vi "BCU诊断标定.vi"(8 "CAN端口":u16(ring), 9 "设备索引号":u16(ring), 10 "CAN卡类型":u32(ring)=21, 11 "Myindex":dbl=1.0) -> (3 "成功":bool)   [LabVIEW 2013] (continued)
                n960 = property on="从板个数" class="DigNum (严格)"("NumText.BGColor"=u32 13816530) -> ()  [unwired: 2 in, 2 out]
                n961 = Select(t=0, s=w1284, f=1) -> (s? t:f=w1283:i32)
                n962 = property on="项目信息" class="Tbl (严格)"("Disabled"=w1283) -> ()  [unwired: 2 in, 2 out]
                n963 = global read "功能码全局.vi" "主板项目信息5"() -> (w1291:bool[])
                n964 = global read "功能码全局.vi" "主板项目信息6"() -> (w1289:bool[])
                n965 = Index Array(array=w1291, index=4 ("索引")) -> (element=w1287:bool)
                n966 = Index Array(array=w1289, index=5 ("索引")) -> (element=w1288:bool)
                n967 = Not(x=w1297) -> (.not. x?=w1296:bool)
              }
              frame "温度起始值" {
                w1333 = 2
                w1335 = FALSE
                n968 = property on="电池实际容量(A)" class="DigNum (严格)"("Disabled"=w1333) -> ()  [unwired: 2 in, 2 out]
                n969 = property on="使用者" class="DigNum (严格)"("Disabled"=w1333) -> ()  [unwired: 2 in, 2 out]
                n970 = property on="SOH(%)" class="DigNum (严格)"("Disabled"=w1333) -> ()  [unwired: 2 in, 2 out]
                n971 = property on="电池额定容量(A)" class="DigNum (严格)"("Disabled"=w1333) -> ()  [unwired: 2 in, 2 out]
                n972 = property on="SOC(%)" class="DigNum (严格)"("Disabled"=w1333) -> ()  [unwired: 2 in, 2 out]
                n973 = local read "从板个数"() -> (w1331:dbl)
                n974 = property on="系统时钟" class="Str"("Disabled"=w1333) -> ()  [unwired: 2 in, 2 out]
                n975 = property on="配置文件版本" class="Str"("Disabled"=w1333) -> ()  [unwired: 2 in, 2 out]
                n976 = property on="车架(牌)号" class="Str"("Disabled"=w1333) -> ()  [unwired: 2 in, 2 out]
                n977 = property on="产品编号" class="Str"("Disabled"=w1333) -> ()  [unwired: 2 in, 2 out]
                n978 = control-ref of="项目信息"() -> (w1332:refnum<vi>)
                n979 = stacked-sequence {
                  tunnel: w1332 -> [w1344 w1347 w1360]
                  tunnel: w1331 -> [w1337 w1346 w1359]
                  frame #0 {
                    n980 = Multiply(x=w1337, y=3.0) -> (x*y=w1339:dbl)
                    n981 = Compound Arithmetic op=ADD(23.0 ("值"), w1339) -> (w1341:dbl)
                    n982 = Bundle(w1341, 0) -> (w1343:cluster{dbl, i32})  [unwired: 1 out]
                    n983 = property class="Tbl (严格)"(reference=w1344, "Index Values"=w1343) -> ()  [unwired: 1 in, 2 out]
                  }
                  frame #1 {
                    n984 = for {
                      N: 10 -> [_]
                      tunnel: w1347 -> [w1357]
                      tunnel: w1346 -> [w1352]
                      i -> [w1351]
                      n985 = Multiply(x=4.0, y=w1352) -> (x*y=w1349:dbl)
                      n986 = Compound Arithmetic op=ADD(24.0 ("值"), w1349, w1351) -> (w1354:dbl)
                      n987 = Bundle(w1354, 0) -> (w1356:cluster{dbl, i32})  [unwired: 1 out]
                      n988 = property class="Tbl (严格)"(reference=w1357, "Active Cell"=w1356, "Cell BG Color"=u32 16448250) -> ()  [unwired: 1 in, 2 out]
                    }
                  }
                  frame #2 {
                    n989 = Increment(x=w1359) -> (x+1=w1358:dbl)
                    n990 = for {
                      N: w1358 -> [_]
                      tunnel: w1360 -> [w1370]
                      tunnel: w1359 -> [w1365]
                      i -> [w1364]
                      n991 = Multiply(x=3.0, y=w1365) -> (x*y=w1362:dbl)
                      n992 = Compound Arithmetic op=ADD(23.0 ("值"), w1362, w1364) -> (w1367:dbl)
                      n993 = Bundle(w1367, 0) -> (w1369:cluster{dbl, i32})  [unwired: 1 out]
                      n994 = property class="Tbl (严格)"(reference=w1370, "Active Cell"=w1369, "Cell BG Color"=u32 6618880) -> ()  [unwired: 1 in, 2 out]
                    }
                  }
                }
                n995 = Select(t=0, s=w1322, f=1) -> (s? t:f=w1321:i32)
                n996 = property on="从板个数" class="DigNum (严格)"("NumText.BGColor"=u32 13816530) -> ()  [unwired: 2 in, 2 out]
                n997 = property on="项目信息" class="Tbl (严格)"("Disabled"=w1321) -> ()  [unwired: 2 in, 2 out]
                n998 = global read "功能码全局.vi" "主板项目信息5"() -> (w1329:bool[])
                n999 = global read "功能码全局.vi" "主板项目信息6"() -> (w1327:bool[])
                n1000 = Index Array(array=w1329, index=5 ("索引")) -> (element=w1326:bool)
                n1001 = Index Array(array=w1327, index=6 ("索引")) -> (element=w1325:bool)
                n1002 = Not(x=w1335) -> (.not. x?=w1334:bool)
              }
              frame "保险位置" {
                w1383 = 2
                w1385 = FALSE
                n1003 = property on="电池实际容量(A)" class="DigNum (严格)"("Disabled"=w1383) -> ()  [unwired: 2 in, 2 out]
                n1004 = property on="使用者" class="DigNum (严格)"("Disabled"=w1383) -> ()  [unwired: 2 in, 2 out]
                n1005 = property on="SOH(%)" class="DigNum (严格)"("Disabled"=w1383) -> ()  [unwired: 2 in, 2 out]
                n1006 = property on="电池额定容量(A)" class="DigNum (严格)"("Disabled"=w1383) -> ()  [unwired: 2 in, 2 out]
                n1007 = property on="SOC(%)" class="DigNum (严格)"("Disabled"=w1383) -> ()  [unwired: 2 in, 2 out]
                n1008 = local read "从板个数"() -> (w1381:dbl)
                n1009 = property on="系统时钟" class="Str"("Disabled"=w1383) -> ()  [unwired: 2 in, 2 out]
                n1010 = property on="配置文件版本" class="Str"("Disabled"=w1383) -> ()  [unwired: 2 in, 2 out]
                n1011 = property on="车架(牌)号" class="Str"("Disabled"=w1383) -> ()  [unwired: 2 in, 2 out]
                n1012 = property on="产品编号" class="Str"("Disabled"=w1383) -> ()  [unwired: 2 in, 2 out]
                n1013 = control-ref of="项目信息"() -> (w1382:refnum<vi>)
                n1014 = stacked-sequence {
                  tunnel: w1382 -> [w1394 w1397]
                  tunnel: w1381 -> [w1387 w1396]
                  frame #0 {
                    n1015 = Multiply(x=w1387, y=4.0) -> (x*y=w1389:dbl)
                    n1016 = Compound Arithmetic op=ADD(24.0 ("值"), w1389) -> (w1391:dbl)
                    n1017 = Bundle(w1391, 0) -> (w1393:cluster{dbl, i32})  [unwired: 1 out]
                    n1018 = property class="Tbl (严格)"(reference=w1394, "Index Values"=w1393) -> ()  [unwired: 1 in, 2 out]
                  }
                  frame #1 {
                    n1019 = for {
                      N: 20 -> [_]
                      tunnel: w1397 -> [w1407]
                      tunnel: w1396 -> [w1402]
                      i -> [w1401]
                      n1020 = Multiply(x=4.0, y=w1402) -> (x*y=w1399:dbl)
                      n1021 = Compound Arithmetic op=ADD(24.0 ("值"), w1399, w1401) -> (w1404:dbl)
                      n1022 = Bundle(w1404, 0) -> (w1406:cluster{dbl, i32})  [unwired: 1 out]
                      n1023 = property class="Tbl (严格)"(reference=w1407, "Active Cell"=w1406, "Cell BG Color"=u32 6618880) -> ()  [unwired: 1 in, 2 out]
                    }
                  }
                }
                n1024 = property on="从板个数" class="DigNum (严格)"("NumText.BGColor"=u32 13816530) -> ()  [unwired: 2 in, 2 out]
                n1025 = Select(t=0, s=w1374, f=1) -> (s? t:f=w1372:i32)
                n1026 = global read "功能码全局.vi" "主板项目信息4"() -> (w1379:bool[])
                n1027 = property on="项目信息" class="Tbl (严格)"("Disabled"=w1372) -> ()  [unwired: 2 in, 2 out]
                n1028 = Index Array(array=w1379, index #1=5 ("索引"), index #2=6 ("索引")) -> (element #1=w1377:bool, element #2=w1376:bool)
                n1029 = Not(x=w1385) -> (.not. x?=w1384:bool)
              }
              frame "SOC" {
                w1418 = 2
                w1420 = FALSE
                n1030 = property on="电池实际容量(A)" class="DigNum (严格)"("Disabled"=w1418) -> ()  [unwired: 2 in, 2 out]
                n1031 = property on="使用者" class="DigNum (严格)"("Disabled"=w1418) -> ()  [unwired: 2 in, 2 out]
                n1032 = property on="SOH(%)" class="DigNum (严格)"("Disabled"=w1418) -> ()  [unwired: 2 in, 2 out]
                n1033 = property on="电池额定容量(A)" class="DigNum (严格)"("Disabled"=w1418) -> ()  [unwired: 2 in, 2 out]
                n1034 = property on="从板个数" class="DigNum (严格)"("NumText.BGColor"=u32 13816530) -> ()  [unwired: 2 in, 2 out]
                n1035 = property on="系统时钟" class="Str"("Disabled"=w1418) -> ()  [unwired: 2 in, 2 out]
                n1036 = property on="配置文件版本" class="Str"("Disabled"=w1418) -> ()  [unwired: 2 in, 2 out]
                n1037 = property on="车架(牌)号" class="Str"("Disabled"=w1418) -> ()  [unwired: 2 in, 2 out]
                n1038 = property on="项目信息" class="Tbl (严格)"("Disabled"=w1418) -> ()  [unwired: 2 in, 2 out]
                n1039 = property on="产品编号" class="Str"("Disabled"=w1418) -> ()  [unwired: 2 in, 2 out]
                n1040 = Select(t=0, s=w1410, f=0) -> (s? t:f=w1409:i32)
                n1041 = property on="SOC(%)" class="DigNum (严格)"("Disabled"=w1409) -> ()  [unwired: 2 in, 2 out]
                n1042 = property on="项目信息2" class="Clust (严格)"("DisabledEnum"=w1409) -> ()  [unwired: 2 in, 2 out]
                n1043 = global read "功能码全局.vi" "主板项目信息7"() -> (w1416:bool[])
                n1044 = Index Array(array=w1416, index #1=2 ("索引"), index #2=5 ("索引")) -> (element #1=w1414:bool, element #2=w1413:bool)
                n1045 = Not(x=w1420) -> (.not. x?=w1419:bool)
              }
              frame "电池额定实际容量" {
                w1432 = 2
                w1434 = FALSE
                n1046 = property on="使用者" class="DigNum (严格)"("Disabled"=w1432) -> ()  [unwired: 2 in, 2 out]
                n1047 = property on="SOH(%)" class="DigNum (严格)"("Disabled"=w1432) -> ()  [unwired: 2 in, 2 out]
                n1048 = property on="SOC(%)" class="DigNum (严格)"("Disabled"=w1432) -> ()  [unwired: 2 in, 2 out]
                n1049 = property on="从板个数" class="DigNum (严格)"("NumText.BGColor"=u32 13816530) -> ()  [unwired: 2 in, 2 out]
                n1050 = property on="系统时钟" class="Str"("Disabled"=w1432) -> ()  [unwired: 2 in, 2 out]
                n1051 = property on="配置文件版本" class="Str"("Disabled"=w1432) -> ()  [unwired: 2 in, 2 out]
                n1052 = property on="车架(牌)号" class="Str"("Disabled"=w1432) -> ()  [unwired: 2 in, 2 out]
                n1053 = property on="项目信息" class="Tbl (严格)"("Disabled"=w1432) -> ()  [unwired: 2 in, 2 out]
                n1054 = property on="产品编号" class="Str"("Disabled"=w1432) -> ()  [unwired: 2 in, 2 out]
                n1055 = Select(t=0, s=w1424, f=1) -> (s? t:f=w1423:i32)
                n1056 = property on="电池实际容量(A)" class="DigNum (严格)"("Disabled"=w1423) -> ()  [unwired: 2 in, 2 out]
                n1057 = property on="电池额定容量(A)" class="DigNum (严格)"("Disabled"=w1423) -> ()  [unwired: 2 in, 2 out]
                n1058 = property on="项目信息2" class="Clust (严格)"("DisabledEnum"=w1423) -> ()  [unwired: 2 in, 2 out]
                n1059 = global read "功能码全局.vi" "主板项目信息7"() -> (w1430:bool[])
                n1060 = Index Array(array=w1430, index #1=3 ("索引"), index #2=6 ("索引")) -> (element #1=w1428:bool, element #2=w1427:bool)
                n1061 = Not(x=w1434) -> (.not. x?=w1433:bool)
              }
              frame "配置文件版本" {
                w1447 = 2
                w1449 = FALSE
                n1062 = property on="使用者" class="DigNum (严格)"("Disabled"=w1447) -> ()  [unwired: 2 in, 2 out]
                n1063 = property on="SOH(%)" class="DigNum (严格)"("Disabled"=w1447) -> ()  [unwired: 2 in, 2 out]
                n1064 = property on="SOC(%)" class="DigNum (严格)"("Disabled"=w1447) -> ()  [unwired: 2 in, 2 out]
                n1065 = property on="电池实际容量(A)" class="DigNum (严格)"("Disabled"=w1447) -> ()  [unwired: 2 in, 2 out]
                n1066 = property on="从板个数" class="DigNum (严格)"("NumText.BGColor"=u32 13816530) -> ()  [unwired: 2 in, 2 out]
                n1067 = property on="电池额定容量(A)" class="DigNum (严格)"("Disabled"=w1447) -> ()  [unwired: 2 in, 2 out]
                n1068 = property on="系统时钟" class="Str"("Disabled"=w1447) -> ()  [unwired: 2 in, 2 out]
                n1069 = property on="车架(牌)号" class="Str"("Disabled"=w1447) -> ()  [unwired: 2 in, 2 out]
                n1070 = property on="项目信息" class="Tbl (严格)"("Disabled"=w1447) -> ()  [unwired: 2 in, 2 out]
                n1071 = property on="产品编号" class="Str"("Disabled"=w1447) -> ()  [unwired: 2 in, 2 out]
                n1072 = Select(t=0, s=w1438, f=1) -> (s? t:f=w1437:i32)
                n1073 = property on="项目信息2" class="Clust (严格)"("DisabledEnum"=w1437) -> ()  [unwired: 2 in, 2 out]
                n1074 = property on="配置文件版本" class="Str"("Disabled"=w1437) -> ()  [unwired: 2 in, 2 out]
                n1075 = global read "功能码全局.vi" "主板项目信息5"() -> (w1445:bool[])
                n1076 = global read "功能码全局.vi" "主板项目信息6"() -> (w1444:bool[])
                n1077 = Index Array(array=w1445, index=6 ("索引")) -> (element=w1442:bool)
                n1078 = Index Array(array=w1444, index=7 ("索引")) -> (element=w1441:bool)
                n1079 = Not(x=w1449) -> (.not. x?=w1448:bool)
              }
              frame "参数修改记录" {
                w1462 = 2
                w1464 = FALSE
                n1080 = property on="SOH(%)" class="DigNum (严格)"("Disabled"=w1462) -> ()  [unwired: 2 in, 2 out]
                n1081 = property on="SOC(%)" class="DigNum (严格)"("Disabled"=w1462) -> ()  [unwired: 2 in, 2 out]
                n1082 = property on="电池实际容量(A)" class="DigNum (严格)"("Disabled"=w1462) -> ()  [unwired: 2 in, 2 out]
                n1083 = property on="电池额定容量(A)" class="DigNum (严格)"("Disabled"=w1462) -> ()  [unwired: 2 in, 2 out]
                n1084 = property on="从板个数" class="DigNum (严格)"("NumText.BGColor"=u32 13816530) -> ()  [unwired: 2 in, 2 out]
                n1085 = property on="系统时钟" class="Str"("Disabled"=w1462) -> ()  [unwired: 2 in, 2 out]
                n1086 = property on="车架(牌)号" class="Str"("Disabled"=w1462) -> ()  [unwired: 2 in, 2 out]
                n1087 = property on="配置文件版本" class="Str"("Disabled"=w1462) -> ()  [unwired: 2 in, 2 out]
                n1088 = property on="项目信息" class="Tbl (严格)"("Disabled"=w1462) -> ()  [unwired: 2 in, 2 out]
                n1089 = property on="产品编号" class="Str"("Disabled"=w1462) -> ()  [unwired: 2 in, 2 out]
                n1090 = Select(t=0, s=w1453, f=1) -> (s? t:f=w1452:i32)
                n1091 = property on="使用者" class="DigNum (严格)"("Disabled"=w1452) -> ()  [unwired: 2 in, 2 out]
                n1092 = property on="项目信息2" class="Clust (严格)"("DisabledEnum"=w1452) -> ()  [unwired: 2 in, 2 out]
                n1093 = global read "功能码全局.vi" "主板项目信息7"() -> (w1459:bool[])
                n1094 = global read "功能码全局.vi" "主板项目信息5"() -> (w1460:bool[])
                n1095 = Index Array(array=w1459, index=0 ("索引")) -> (element=w1457:bool)
                n1096 = Index Array(array=w1460, index=7 ("索引")) -> (element=w1456:bool)
                n1097 = Not(x=w1464) -> (.not. x?=w1463:bool)
              }
              frame "车牌号" {
                w1477 = 2
                w1479 = FALSE
                n1098 = property on="SOH(%)" class="DigNum (严格)"("Disabled"=w1477) -> ()  [unwired: 2 in, 2 out]
                n1099 = property on="使用者" class="DigNum (严格)"("Disabled"=w1477) -> ()  [unwired: 2 in, 2 out]
                n1100 = property on="SOC(%)" class="DigNum (严格)"("Disabled"=w1477) -> ()  [unwired: 2 in, 2 out]
                n1101 = property on="电池实际容量(A)" class="DigNum (严格)"("Disabled"=w1477) -> ()  [unwired: 2 in, 2 out]
                n1102 = property on="电池额定容量(A)" class="DigNum (严格)"("Disabled"=w1477) -> ()  [unwired: 2 in, 2 out]
                n1103 = property on="从板个数" class="DigNum (严格)"("NumText.BGColor"=u32 13816530) -> ()  [unwired: 2 in, 2 out]
                n1104 = property on="系统时钟" class="Str"("Disabled"=w1477) -> ()  [unwired: 2 in, 2 out]
                n1105 = property on="配置文件版本" class="Str"("Disabled"=w1477) -> ()  [unwired: 2 in, 2 out]
                n1106 = property on="项目信息" class="Tbl (严格)"("Disabled"=w1477) -> ()  [unwired: 2 in, 2 out]
                n1107 = property on="产品编号" class="Str"("Disabled"=w1477) -> ()  [unwired: 2 in, 2 out]
                n1108 = Select(t=0, s=w1468, f=1) -> (s? t:f=w1467:i32)
                n1109 = property on="车架(牌)号" class="Str"("Disabled"=w1467) -> ()  [unwired: 2 in, 2 out]
                n1110 = property on="项目信息2" class="Clust (严格)"("DisabledEnum"=w1467) -> ()  [unwired: 2 in, 2 out]
                n1111 = global read "功能码全局.vi" "主板项目信息7"() -> (w1474:bool[])
                n1112 = global read "功能码全局.vi" "主板项目信息6"() -> (w1475:bool[])
                n1113 = Index Array(array=w1474, index=1 ("索引")) -> (element=w1472:bool)
                n1114 = Index Array(array=w1475, index=0 ("索引")) -> (element=w1471:bool)
                n1115 = Not(x=w1479) -> (.not. x?=w1478:bool)
              }
              frame "SOH" {
                w1491 = 2
                w1493 = FALSE
                n1116 = property on="使用者" class="DigNum (严格)"("Disabled"=w1491) -> ()  [unwired: 2 in, 2 out]
                n1117 = property on="SOC(%)" class="DigNum (严格)"("Disabled"=w1491) -> ()  [unwired: 2 in, 2 out]
                n1118 = property on="电池实际容量(A)" class="DigNum (严格)"("Disabled"=w1491) -> ()  [unwired: 2 in, 2 out]
                n1119 = property on="电池额定容量(A)" class="DigNum (严格)"("Disabled"=w1491) -> ()  [unwired: 2 in, 2 out]
                n1120 = property on="从板个数" class="DigNum (严格)"("NumText.BGColor"=u32 13816530) -> ()  [unwired: 2 in, 2 out]
                n1121 = property on="系统时钟" class="Str"("Disabled"=w1491) -> ()  [unwired: 2 in, 2 out]
                n1122 = property on="配置文件版本" class="Str"("Disabled"=w1491) -> ()  [unwired: 2 in, 2 out]
                n1123 = property on="项目信息" class="Tbl (严格)"("Disabled"=w1491) -> ()  [unwired: 2 in, 2 out]
                n1124 = property on="产品编号" class="Str"("Disabled"=w1491) -> ()  [unwired: 2 in, 2 out]
                n1125 = property on="车架(牌)号" class="Str"("Disabled"=w1491) -> ()  [unwired: 2 in, 2 out]
                n1126 = Select(t=0, s=w1483, f=1) -> (s? t:f=w1482:i32)
                n1127 = property on="项目信息2" class="Clust (严格)"("DisabledEnum"=w1482) -> ()  [unwired: 2 in, 2 out]
                n1128 = property on="SOH(%)" class="DigNum (严格)"("Disabled"=w1482) -> ()  [unwired: 2 in, 2 out]
                n1129 = global read "功能码全局.vi" "主板项目信息7"() -> (w1490:bool[])
                n1130 = Index Array(array=w1490, index #1=4 ("索引"), index #2=7 ("索引")) -> (element #1=w1487:bool, element #2=w1486:bool)
                n1131 = Not(x=w1493) -> (.not. x?=w1492:bool)
              }
              frame "SOC过低(2)", "SOC过高(2)", "SOH过低(2)", "充电电流过高(2)", "单体电压过低(2)", "单体电压过高(2)", "单组电压不均衡(2)", "单组温度不均衡(2)", "二级故障阀值", "放电电流过高(2)", "极柱温度过高(2)", "内阻过大(2)", "温度过低(2)", "温度过高(2)", "整组电压不均衡(2)", "整组温度不均衡(2)", "总电压过低(2)", "总电压过高(2)" {
                w1505 = FALSE
                n1132 = property on="从板个数" class="DigNum (严格)"("NumText.BGColor"=u32 13816530) -> ()  [unwired: 2 in, 2 out]
                n1133 = Select(t=0, s=w1497, f=1) -> (s? t:f=w1496:i32)
                n1134 = property on="一级故障 2" class="Clust (严格)"("DisabledEnum"=w1496) -> ()  [unwired: 2 in, 2 out]
                n1135 = global read "功能码全局.vi" "主板故障阀值9"() -> (w1503:bool[])
                n1136 = Index Array(array=w1503, index #1=3 ("索引"), index #2=6 ("索引")) -> (element #1=w1501:bool, element #2=w1500:bool)
                n1137 = Not(x=w1505) -> (.not. x?=w1506:bool)
              }
              frame "SOC过低(3)", "SOC过高(3)", "SOH过低(3)", "充电电流过高(3)", "单体电压过低(3)", "单体电压过高(3)", "单组电压不均衡(3)", "单组温度不均衡(3)", "放电电流过高(3)", "极柱温度过高(3)", "内阻过大(3)", "三级故障阀值", "温度过低(3)", "温度过高(3)", "整组电压不均衡(3)", "整组温度不均衡(3)", "总电压过低(3)", "总电压过高(3)" {
                w1519 = FALSE
                n1138 = property on="从板个数" class="DigNum (严格)"("NumText.BGColor"=u32 13816530) -> ()  [unwired: 2 in, 2 out]
                n1139 = Select(t=0, s=w1510, f=1) -> (s? t:f=w1509:i32)
                n1140 = property on="一级故障 3" class="Clust (严格)"("DisabledEnum"=w1509) -> ()  [unwired: 2 in, 2 out]
                n1141 = global read "功能码全局.vi" "主板故障阀值9"() -> (w1516:bool[])
                n1142 = Index Array(array=w1516, index #1=4 ("索引"), index #2=7 ("索引")) -> (element #1=w1514:bool, element #2=w1513:bool)
                n1143 = Not(x=w1519) -> (.not. x?=w1518:bool)
              }
              frame "SOC过低", "SOC过高", "SOH过低", "充电电流过高", "单体电压过低", "单体电压过高", "单组电压不均衡", "单组温度不均衡", "放电电流过高", "极柱温度过高", "内阻过大", "温度过低", "温度过高", "一级故障阀值", "整组电压不均衡", "整组温度不均衡", "总电压过低", "总电压过高" {
                w1532 = FALSE
                n1144 = Select(t=0, s=w1523, f=1) -> (s? t:f=w1522:i32)
                n1145 = property on="从板个数" class="DigNum (严格)"("NumText.BGColor"=u32 13816530) -> ()  [unwired: 2 in, 2 out]
                n1146 = property on="一级故障" class="Clust (严格)"("DisabledEnum"=w1522) -> ()  [unwired: 2 in, 2 out]
                n1147 = global read "功能码全局.vi" "主板故障阀值9"() -> (w1529:bool[])
                n1148 = Index Array(array=w1529, index #1=2 ("索引"), index #2=5 ("索引")) -> (element #1=w1527:bool, element #2=w1526:bool)
                n1149 = Not(x=w1532) -> (.not. x?=w1531:bool)
              }
              frame "充电控制参数", "电流步长", "最大允许充电电流", "最大允许充电温度", "最大允许单体电压", "最大允许总电压", "最小允许充电电流", "最小允许充电温度", "最小允许单体电压" {
                w1535 = 2
                w1546 = FALSE
                n1150 = property on="从板个数" class="DigNum (严格)"("NumText.BGColor"=u32 13816530) -> ()  [unwired: 2 in, 2 out]
                n1151 = property on="风机开启温度" class="DigNum (严格)"("Disabled"=w1535) -> ()  [unwired: 2 in, 2 out]
                n1152 = property on="风机关闭温度" class="DigNum (严格)"("Disabled"=w1535) -> ()  [unwired: 2 in, 2 out]
                n1153 = property on="加热开启温度" class="DigNum (严格)"("Disabled"=w1535) -> ()  [unwired: 2 in, 2 out]
                n1154 = property on="加热关闭温度" class="DigNum (严格)"("Disabled"=w1535) -> ()  [unwired: 2 in, 2 out]
                n1155 = property on="风机开启温差" class="DigNum (严格)"("Disabled"=w1535) -> ()  [unwired: 2 in, 2 out]
                n1156 = property on="风机关闭温差" class="DigNum (严格)"("Disabled"=w1535) -> ()  [unwired: 2 in, 2 out]
                n1157 = property on="加热控制参数" class="Clust (严格)"("DisabledEnum"=w1535) -> ()  [unwired: 2 in, 2 out]
                n1158 = Select(t=0, s=w1537, f=1) -> (s? t:f=w1536:i32)
                n1159 = property on="最大允许总电压" class="DigNum (严格)"("Disabled"=w1536) -> ()  [unwired: 2 in, 2 out]
                n1160 = property on="最大允许充电温度" class="DigNum (严格)"("Disabled"=w1536) -> ()  [unwired: 2 in, 2 out]
                n1161 = property on="最小允许充电温度" class="DigNum (严格)"("Disabled"=w1536) -> ()  [unwired: 2 in, 2 out]
                n1162 = property on="电流步长" class="DigNum (严格)"("Disabled"=w1536) -> ()  [unwired: 2 in, 2 out]
                n1163 = property on="最大允许单体电压" class="DigNum (严格)"("Disabled"=w1536) -> ()  [unwired: 2 in, 2 out]
                n1164 = property on="最小允许单体电压" class="DigNum (严格)"("Disabled"=w1536) -> ()  [unwired: 2 in, 2 out]
                n1165 = property on="最大允许充电电流" class="DigNum (严格)"("Disabled"=w1536) -> ()  [unwired: 2 in, 2 out]
                n1166 = property on="最小允许充电电流" class="DigNum (严格)"("Disabled"=w1536) -> ()  [unwired: 2 in, 2 out]
                n1167 = global read "功能码全局.vi" "主板控制类信息10"() -> (w1543:bool[])
                n1168 = Index Array(array=w1543, index #1=5 ("索引"), index #2=7 ("索引")) -> (element #1=w1541:bool, element #2=w1540:bool)
                n1169 = Not(x=w1546) -> (.not. x?=w1545:bool)
              }
              frame "风机关闭温差", "风机关闭温度", "风机开启温差", "风机开启温度", "加热关闭温差", "加热关闭温度", "加热开启温度", "加热控制参数" {
                w1558 = 2
                w1560 = FALSE
                n1170 = Select(t=0, s=w1550, f=1) -> (s? t:f=w1549:i32)
                n1171 = property on="从板个数" class="DigNum (严格)"("NumText.BGColor"=u32 13816530) -> ()  [unwired: 2 in, 2 out]
                n1172 = property on="加热控制参数" class="Clust (严格)"("DisabledEnum"=w1549) -> ()  [unwired: 2 in, 2 out]
                n1173 = property on="风机开启温度" class="DigNum (严格)"("Disabled"=w1549) -> ()  [unwired: 2 in, 2 out]
                n1174 = property on="风机关闭温度" class="DigNum (严格)"("Disabled"=w1549) -> ()  [unwired: 2 in, 2 out]
                n1175 = property on="加热开启温度" class="DigNum (严格)"("Disabled"=w1549) -> ()  [unwired: 2 in, 2 out]
                n1176 = property on="加热关闭温度" class="DigNum (严格)"("Disabled"=w1549) -> ()  [unwired: 2 in, 2 out]
                n1177 = property on="风机开启温差" class="DigNum (严格)"("Disabled"=w1549) -> ()  [unwired: 2 in, 2 out]
                n1178 = property on="风机关闭温差" class="DigNum (严格)"("Disabled"=w1549) -> ()  [unwired: 2 in, 2 out]
                n1179 = property on="最大允许总电压" class="DigNum (严格)"("Disabled"=w1558) -> ()  [unwired: 2 in, 2 out]
                n1180 = property on="最大允许充电温度" class="DigNum (严格)"("Disabled"=w1558) -> ()  [unwired: 2 in, 2 out]
                n1181 = property on="最小允许充电温度" class="DigNum (严格)"("Disabled"=w1558) -> ()  [unwired: 2 in, 2 out]
                n1182 = property on="电流步长" class="DigNum (严格)"("Disabled"=w1558) -> ()  [unwired: 2 in, 2 out]
                n1183 = property on="最大允许单体电压" class="DigNum (严格)"("Disabled"=w1558) -> ()  [unwired: 2 in, 2 out]
                n1184 = property on="最小允许单体电压" class="DigNum (严格)"("Disabled"=w1558) -> ()  [unwired: 2 in, 2 out]
                n1185 = property on="最大允许充电电流" class="DigNum (严格)"("Disabled"=w1558) -> ()  [unwired: 2 in, 2 out]
                n1186 = property on="最小允许充电电流" class="DigNum (严格)"("Disabled"=w1558) -> ()  [unwired: 2 in, 2 out]
                n1187 = global read "功能码全局.vi" "主板控制类信息10"() -> (w1556:bool[])
                n1188 = Index Array(array=w1556, index #1=4 ("索引"), index #2=6 ("索引")) -> (element #1=w1554:bool, element #2=w1553:bool)
                n1189 = Not(x=w1560) -> (.not. x?=w1559:bool)
              }
              frame "电池信息" {
                w1573 = FALSE
                n1190 = Select(t=0, s=w1564, f=1) -> (s? t:f=w1563:i32)
                n1191 = property on="电池串联" class="DigNum (严格)"("Disabled"=w1563) -> ()  [unwired: 2 in, 2 out]
                n1192 = property on="电池并联" class="DigNum (严格)"("Disabled"=w1563) -> ()  [unwired: 2 in, 2 out]
                n1193 = property on="电池包额定容量" class="DigNum (严格)"("Disabled"=w1563) -> ()  [unwired: 2 in, 2 out]
                n1194 = property on="电池包额定能量(kWh)" class="DigNum (严格)"("Disabled"=w1563) -> ()  [unwired: 2 in, 2 out]
                n1195 = property on="电池包额定总电压" class="DigNum (严格)"("Disabled"=w1563) -> ()  [unwired: 2 in, 2 out]
                n1196 = property on="实际容量" class="DigNum (严格)"("Disabled"=w1563) -> ()  [unwired: 2 in, 2 out]
                n1197 = property on="电池包组号" class="Str"("Disabled"=w1563) -> ()  [unwired: 2 in, 2 out]
                n1198 = property on="电池生产日期" class="Str"("Disabled"=w1563) -> ()  [unwired: 2 in, 2 out]
                n1199 = property on="电池厂家" class="Str"("Disabled"=w1563) -> ()  [unwired: 2 in, 2 out]
                n1200 = property on="电池类型" class="Str"("Disabled"=w1563) -> ()  [unwired: 2 in, 2 out]
                n1201 = property on="累计充电总安时" class="DigNum (严格)"("Disabled"=w1563) -> ()  [unwired: 2 in, 2 out]
                n1202 = property on="累计放电总安时" class="DigNum (严格)"("Disabled"=w1563) -> ()  [unwired: 2 in, 2 out]
                n1203 = property on="电池放空次数" class="DigNum (严格)"("Disabled"=w1563) -> ()  [unwired: 2 in, 2 out]
                n1204 = property on="电池充满次数" class="DigNum (严格)"("Disabled"=w1563) -> ()  [unwired: 2 in, 2 out]
                n1205 = property on="电池充电次数" class="DigNum (严格)"("Disabled"=w1563) -> ()  [unwired: 2 in, 2 out]
                n1206 = property on="电池信息" class="Clust (严格)"("DisabledEnum"=w1563) -> ()  [unwired: 2 in, 2 out]
                n1207 = global read "功能码全局.vi" "主板版本号11"() -> (w1570:bool[])
                n1208 = property on="从板个数" class="DigNum (严格)"("NumText.BGColor"=u32 13816530) -> ()  [unwired: 2 in, 2 out]
                n1209 = Index Array(array=w1570, index #1=0 ("索引"), index #2=1 ("索引")) -> (element #1=w1568:bool, element #2=w1567:bool)
                n1210 = Not(x=w1573) -> (.not. x?=w1572:bool)
              }
              frame "电池信息1" {
                w1585 = 2
                w1587 = FALSE
                n1211 = Select(t=0, s=w1577, f=1) -> (s? t:f=w1576:i32)
                n1212 = property on="电池信息" class="Clust (严格)"("DisabledEnum"=w1576) -> ()  [unwired: 2 in, 2 out]
                n1213 = property on="电池生产日期" class="Str"("Disabled"=w1576) -> ()  [unwired: 2 in, 2 out]
                n1214 = property on="电池厂家" class="Str"("Disabled"=w1576) -> ()  [unwired: 2 in, 2 out]
                n1215 = property on="电池类型" class="Str"("Disabled"=w1576) -> ()  [unwired: 2 in, 2 out]
                n1216 = property on="电池串联" class="DigNum (严格)"("Disabled"=w1576) -> ()  [unwired: 2 in, 2 out]
                n1217 = property on="电池并联" class="DigNum (严格)"("Disabled"=w1576) -> ()  [unwired: 2 in, 2 out]
                n1218 = property on="电池包额定容量" class="DigNum (严格)"("Disabled"=w1576) -> ()  [unwired: 2 in, 2 out]
                n1219 = property on="电池包额定能量(kWh)" class="DigNum (严格)"("Disabled"=w1576) -> ()  [unwired: 2 in, 2 out]
                n1220 = property on="电池包额定总电压" class="DigNum (严格)"("Disabled"=w1576) -> ()  [unwired: 2 in, 2 out]
                n1221 = property on="实际容量" class="DigNum (严格)"("Disabled"=w1576) -> ()  [unwired: 2 in, 2 out]
                n1222 = property on="累计充电总安时" class="DigNum (严格)"("Disabled"=w1585) -> ()  [unwired: 2 in, 2 out]
                n1223 = property on="累计放电总安时" class="DigNum (严格)"("Disabled"=w1585) -> ()  [unwired: 2 in, 2 out]
                n1224 = property on="电池放空次数" class="DigNum (严格)"("Disabled"=w1585) -> ()  [unwired: 2 in, 2 out]
                n1225 = property on="电池充满次数" class="DigNum (严格)"("Disabled"=w1585) -> ()  [unwired: 2 in, 2 out]
                n1226 = property on="电池充电次数" class="DigNum (严格)"("Disabled"=w1585) -> ()  [unwired: 2 in, 2 out]
                n1227 = property on="从板个数" class="DigNum (严格)"("NumText.BGColor"=u32 13816530) -> ()  [unwired: 2 in, 2 out]
                n1228 = property on="电池包组号" class="Str"("Disabled"=w1585) -> ()  [unwired: 2 in, 2 out]
                n1229 = global read "功能码全局.vi" "主板版本号11"() -> (w1583:bool[])
                n1230 = Index Array(array=w1583, index #1=0 ("索引"), index #2=1 ("索引")) -> (element #1=w1581:bool, element #2=w1580:bool)
                n1231 = Not(x=w1587) -> (.not. x?=w1586:bool)
              }
              frame "电池包组号" {
                w1599 = 2
                w1601 = FALSE
                n1232 = property on="电池生产日期" class="Str"("Disabled"=w1599) -> ()  [unwired: 2 in, 2 out]
                n1233 = property on="电池厂家" class="Str"("Disabled"=w1599) -> ()  [unwired: 2 in, 2 out]
                n1234 = property on="电池类型" class="Str"("Disabled"=w1599) -> ()  [unwired: 2 in, 2 out]
                n1235 = property on="电池串联" class="DigNum (严格)"("Disabled"=w1599) -> ()  [unwired: 2 in, 2 out]
                n1236 = property on="电池并联" class="DigNum (严格)"("Disabled"=w1599) -> ()  [unwired: 2 in, 2 out]
                n1237 = property on="电池包额定容量" class="DigNum (严格)"("Disabled"=w1599) -> ()  [unwired: 2 in, 2 out]
                n1238 = property on="电池包额定能量(kWh)" class="DigNum (严格)"("Disabled"=w1599) -> ()  [unwired: 2 in, 2 out]
                n1239 = property on="电池包额定总电压" class="DigNum (严格)"("Disabled"=w1599) -> ()  [unwired: 2 in, 2 out]
                n1240 = property on="实际容量" class="DigNum (严格)"("Disabled"=w1599) -> ()  [unwired: 2 in, 2 out]
                n1241 = property on="从板个数" class="DigNum (严格)"("NumText.BGColor"=u32 13816530) -> ()  [unwired: 2 in, 2 out]
                n1242 = property on="累计充电总安时" class="DigNum (严格)"("Disabled"=w1599) -> ()  [unwired: 2 in, 2 out]
                n1243 = property on="累计放电总安时" class="DigNum (严格)"("Disabled"=w1599) -> ()  [unwired: 2 in, 2 out]
                n1244 = property on="电池放空次数" class="DigNum (严格)"("Disabled"=w1599) -> ()  [unwired: 2 in, 2 out]
                n1245 = property on="电池充满次数" class="DigNum (严格)"("Disabled"=w1599) -> ()  [unwired: 2 in, 2 out]
                n1246 = property on="电池充电次数" class="DigNum (严格)"("Disabled"=w1599) -> ()  [unwired: 2 in, 2 out]
                n1247 = Select(t=0, s=w1591, f=1) -> (s? t:f=w1590:i32)
                n1248 = property on="电池包组号" class="Str"("Disabled"=w1590) -> ()  [unwired: 2 in, 2 out]
                n1249 = property on="电池信息" class="Clust (严格)"("DisabledEnum"=w1590) -> ()  [unwired: 2 in, 2 out]
                n1250 = global read "功能码全局.vi" "主板版本号11"() -> (w1597:bool[])
                n1251 = Index Array(array=w1597, index #1=0 ("索引"), index #2=1 ("索引")) -> (element #1=w1595:bool, element #2=w1594:bool)
                n1252 = Not(x=w1601) -> (.not. x?=w1600:bool)
              }
              frame "充放电安时" {
                w1613 = 2
                w1615 = FALSE
                n1253 = property on="电池生产日期" class="Str"("Disabled"=w1613) -> ()  [unwired: 2 in, 2 out]
                n1254 = property on="电池厂家" class="Str"("Disabled"=w1613) -> ()  [unwired: 2 in, 2 out]
                n1255 = property on="电池类型" class="Str"("Disabled"=w1613) -> ()  [unwired: 2 in, 2 out]
                n1256 = property on="电池串联" class="DigNum (严格)"("Disabled"=w1613) -> ()  [unwired: 2 in, 2 out]
                n1257 = property on="电池并联" class="DigNum (严格)"("Disabled"=w1613) -> ()  [unwired: 2 in, 2 out]
                n1258 = property on="电池包额定容量" class="DigNum (严格)"("Disabled"=w1613) -> ()  [unwired: 2 in, 2 out]
                n1259 = property on="电池包额定能量(kWh)" class="DigNum (严格)"("Disabled"=w1613) -> ()  [unwired: 2 in, 2 out]
                n1260 = property on="电池包额定总电压" class="DigNum (严格)"("Disabled"=w1613) -> ()  [unwired: 2 in, 2 out]
                n1261 = property on="实际容量" class="DigNum (严格)"("Disabled"=w1613) -> ()  [unwired: 2 in, 2 out]
                n1262 = property on="从板个数" class="DigNum (严格)"("NumText.BGColor"=u32 13816530) -> ()  [unwired: 2 in, 2 out]
                n1263 = Select(t=0, s=w1605, f=1) -> (s? t:f=w1604:i32)
                n1264 = property on="电池放空次数" class="DigNum (严格)"("Disabled"=w1613) -> ()  [unwired: 2 in, 2 out]
                n1265 = property on="电池充满次数" class="DigNum (严格)"("Disabled"=w1613) -> ()  [unwired: 2 in, 2 out]
                n1266 = property on="电池充电次数" class="DigNum (严格)"("Disabled"=w1613) -> ()  [unwired: 2 in, 2 out]
                n1267 = property on="电池包组号" class="Str"("Disabled"=w1613) -> ()  [unwired: 2 in, 2 out]
                n1268 = property on="累计充电总安时" class="DigNum (严格)"("Disabled"=w1604) -> ()  [unwired: 2 in, 2 out]
                n1269 = property on="累计放电总安时" class="DigNum (严格)"("Disabled"=w1604) -> ()  [unwired: 2 in, 2 out]
                n1270 = property on="电池信息" class="Clust (严格)"("DisabledEnum"=w1604) -> ()  [unwired: 2 in, 2 out]
                n1271 = global read "功能码全局.vi" "主板版本号11"() -> (w1611:bool[])
                n1272 = Index Array(array=w1611, index #1=0 ("索引"), index #2=1 ("索引")) -> (element #1=w1609:bool, element #2=w1608:bool)
                n1273 = Not(x=w1615) -> (.not. x?=w1614:bool)
              }
              frame "电池充放电次数" {
                w1627 = 2
                w1629 = FALSE
                n1274 = property on="从板个数" class="DigNum (严格)"("NumText.BGColor"=u32 13816530) -> ()  [unwired: 2 in, 2 out]
                n1275 = property on="电池生产日期" class="Str"("Disabled"=w1627) -> ()  [unwired: 2 in, 2 out]
                n1276 = property on="电池厂家" class="Str"("Disabled"=w1627) -> ()  [unwired: 2 in, 2 out]
                n1277 = property on="电池类型" class="Str"("Disabled"=w1627) -> ()  [unwired: 2 in, 2 out]
                n1278 = property on="电池串联" class="DigNum (严格)"("Disabled"=w1627) -> ()  [unwired: 2 in, 2 out]
                n1279 = property on="电池并联" class="DigNum (严格)"("Disabled"=w1627) -> ()  [unwired: 2 in, 2 out]
                n1280 = property on="电池包额定容量" class="DigNum (严格)"("Disabled"=w1627) -> ()  [unwired: 2 in, 2 out]
                n1281 = property on="电池包额定能量(kWh)" class="DigNum (严格)"("Disabled"=w1627) -> ()  [unwired: 2 in, 2 out]
                n1282 = property on="电池包额定总电压" class="DigNum (严格)"("Disabled"=w1627) -> ()  [unwired: 2 in, 2 out]
                n1283 = property on="实际容量" class="DigNum (严格)"("Disabled"=w1627) -> ()  [unwired: 2 in, 2 out]
                n1284 = Select(t=0, s=w1619, f=1) -> (s? t:f=w1618:i32)
                n1285 = property on="电池放空次数" class="DigNum (严格)"("Disabled"=w1618) -> ()  [unwired: 2 in, 2 out]
                n1286 = property on="电池充满次数" class="DigNum (严格)"("Disabled"=w1618) -> ()  [unwired: 2 in, 2 out]
                n1287 = property on="电池充电次数" class="DigNum (严格)"("Disabled"=w1618) -> ()  [unwired: 2 in, 2 out]
                n1288 = property on="累计充电总安时" class="DigNum (严格)"("Disabled"=w1627) -> ()  [unwired: 2 in, 2 out]
                n1289 = property on="累计放电总安时" class="DigNum (严格)"("Disabled"=w1627) -> ()  [unwired: 2 in, 2 out]
                n1290 = property on="电池信息" class="Clust (严格)"("DisabledEnum"=w1618) -> ()  [unwired: 2 in, 2 out]
                n1291 = property on="电池包组号" class="Str"("Disabled"=w1627) -> ()  [unwired: 2 in, 2 out]
                n1292 = global read "功能码全局.vi" "主板版本号11"() -> (w1625:bool[])
                n1293 = Index Array(array=w1625, index #1=0 ("索引"), index #2=1 ("索引")) -> (element #1=w1623:bool, element #2=w1622:bool)
                n1294 = Not(x=w1629) -> (.not. x?=w1628:bool)
              }
              frame "假", Default {
                w1634 = FALSE
                n1295 = Not(x=w1634) -> (.not. x?=w1633:bool)
              }
            }
            n1296 = property on="单个读取" class="Bool (严格)"("Visible"=w1117) -> ()  [unwired: 2 in, 2 out]
            n1297 = property on="单个写入" class="Bool (严格)"("Visible"=w1116) -> ()  [unwired: 2 in, 2 out]
            n1298 = local write "1"(w1124) -> ()
            n1299 = local write "1 2"(w1123) -> ()
            n1300 = local write "1 3"(w1122) -> ()
            n1301 = local write "1 4"(w1121) -> ()
            n1302 = local write "1 5"(w1120) -> ()
            n1303 = local write "1 11"(w1119) -> ()
            n1304 = local write "主板2"(w1125) -> ()
          }
          event "从板选项": Mouse Down {
            n1305 = event-data() -> ("CtlRef"=w1649:refnum<vi>)  [unwired: 8 out]
            n1306 = property class="Tree (严格)"(reference=w1649) -> ("Value"=w1648:string)  [unwired: 1 in, 2 out]
            n1307 = global read "功能码全局.vi" "主板监控2"() -> (w1639:bool[])
            n1308 = Index Array(array=w1639, index=6 ("索引")) -> (element=w1637:bool)
            n1309 = case shown="\"温度个数\"" w1648 {
              tunnel: [T21."从板信息" ("等级 2") T21."从板信息" ("等级 2") T21."从板信息" ("等级 2") T21."从板信息" ("等级 2") T21."从板信息" ("等级 2") T21."从板信息" ("等级 2") T21."从板信息" ("等级 2") T21."一级故障阀值" ("等级 2") T21."二级故障阀值" ("等级 2") T21."三级故障阀值" ("等级 2") T21."快换参数" ("等级 2") T21."快换参数" ("等级 2") T21."快换参数" ("等级 2") T21."快换参数" ("等级 2") T21."快换参数" ("等级 2") T21."快换参数" ("等级 2") T21."快换参数" ("等级 2") T21."快换参数" ("等级 2") T14."均衡参数" ("等级 2") T14."均衡参数" ("等级 2") T14."均衡参数" ("等级 2") T21."从板信息" ("等级 2")] -> w1647
              tunnel: [w1660 w1670 w1684 w1699 w1734 w1771 w1808 w1832 w1845 w1858 w1871 w1897 w1911 w1927 w1944 w1961 w1979 w1998 w2015 w2028 w2042 w2057] -> w1646
              tunnel: [w1652 w1662 w1672 w1686 w1721 w1758 w1795 w1843 w1845 w1858 w1871 w1897 w1911 w1927 w1944 w1961 w1979 w1998 w2015 w2028 w2042 w2056] -> w1645
              tunnel: [w1652 w1662 w1672 w1686 w1721 w1758 w1795 w1832 w1856 w1858 w1871 w1897 w1911 w1927 w1944 w1961 w1979 w1998 w2015 w2028 w2042 w2056] -> w1644
              tunnel: [w1652 w1662 w1672 w1686 w1721 w1758 w1795 w1832 w1845 w1869 w1871 w1897 w1911 w1927 w1944 w1961 w1979 w1998 w2015 w2028 w2042 w2056] -> w1643
              tunnel: [w1652 w1662 w1672 w1686 w1721 w1758 w1795 w1832 w1845 w1858 w1895 w1909 w1925 w1942 w1959 w1977 w1996 w2013 w2015 w2028 w2042 w2056] -> w1642
              tunnel: [w1657 w1663 w1679 w1693 w1728 w1765 w1802 w1839 w1852 w1865 w1880 w1902 w1917 w1931 w1949 w1964 w1984 w2002 w2018 w2032 w2047 w2056] -> w1641
              tunnel: [w1654 w1663 w1678 w1692 w1727 w1764 w1801 w1838 w1851 w1864 w1872 w1901 w1916 w1930 w1950 w1965 w1983 w2001 w2017 w2031 w2046 w2056] -> w1640
              tunnel: w1637 -> [_ w1667 w1675 w1689 w1724 w1761 w1798 w1834 w1848 w1861 w1892 w1905 w1920 w1935 w1953 w1969 w1987 w2006 w2021 w2035 w2049 _]
              tunnel: [w1652 w1662 w1672 w1686 w1721 w1758 w1795 w1832 w1845 w1858 w1871 w1897 w1911 w1927 w1944 w1961 w1979 w1998 w2016 w2029 w2043 w2056] -> w1636
              frame "从板号" {
                w1659 = 2
                w1652 = FALSE ("1 6")
                n1310 = property on="项目信息 2" class="Tbl (严格)"("Disabled"=w1659) -> ()  [unwired: 2 in, 2 out]
                n1311 = property on="加热控制参数" class="Clust (严格)"("Disabled"=w1659) -> ()  [unwired: 2 in, 2 out]
                n1312 = property on="从板号" class="DigNum (严格)"("NumText.BGColor"=u32 6618880) -> ()  [unwired: 2 in, 2 out]
                n1313 = global read "功能码全局.vi" "16"() -> (w1656:bool[])
                n1314 = Index Array(array=w1656, index #1=4 ("索引"), index #2=6 ("索引")) -> (element #1=w1657:bool, element #2=w1654:bool)
                n1315 = Not(x=w1652) -> (.not. x?=w1660:bool)
              }
              frame "从板信息" {
                w1662 = FALSE ("1 6")
                n1316 = Select(t=0, s=w1667, f=1) -> (s? t:f=w1666:i32)
                n1317 = property on="从板号" class="DigNum (严格)"("NumText.BGColor"=u32 16777215) -> ()  [unwired: 2 in, 2 out]
                n1318 = property on="项目信息 2" class="Tbl (严格)"("Disabled"=w1666) -> ()  [unwired: 2 in, 2 out]
                n1319 = property on="加热控制参数" class="Clust (严格)"("Disabled"=w1666) -> ()  [unwired: 2 in, 2 out]
                n1320 = Not(x=w1662) -> (.not. x?=w1670:bool)
                n1321 = local read "从板项目信息"() -> (w1664:bool)
                n1322 = Not(x=w1664) -> (.not. x?=w1663:bool)
              }
              frame "风机关闭温差", "风机关闭温度", "风机开启温差", "风机开启温度", "加热关闭温差", "加热关闭温度", "加热开启温度", "加热控制参数" {
                w1672 = FALSE ("1 6")
                n1323 = property on="从板号" class="DigNum (严格)"("NumText.BGColor"=u32 16777215) -> ()  [unwired: 2 in, 2 out]
                n1324 = Select(t=0, s=w1675, f=1) -> (s? t:f=w1674:i32)
                n1325 = property on="项目信息 2" class="Tbl (严格)"("Disabled"=2) -> ()  [unwired: 2 in, 2 out]
                n1326 = property on="加热控制参数" class="Clust (严格)"("Disabled"=w1674) -> ()  [unwired: 2 in, 2 out]
                n1327 = global read "功能码全局.vi" "16"() -> (w1681:bool[])
                n1328 = Index Array(array=w1681, index #1=5 ("索引"), index #2=7 ("索引")) -> (element #1=w1679:bool, element #2=w1678:bool)
                n1329 = Not(x=w1672) -> (.not. x?=w1684:bool)
              }
              frame "电压个数" {
                w1686 = FALSE ("1 6")
                n1330 = property on="从板号" class="DigNum (严格)"("NumText.BGColor"=u32 16777215) -> ()  [unwired: 2 in, 2 out]
                n1331 = control-ref of="项目信息 2"() -> (w1697:refnum<vi>)
                n1332 = stacked-sequence {
                  tunnel: w1697 -> [w1704 w1706 w1715]
                  frame #0 {
                    n1333 = Bundle(0, 0) -> (w1703:cluster{i32, i32})  [unwired: 1 out]
                    n1334 = property class="Tbl (严格)"(reference=w1704, "Index Values"=w1703) -> ()  [unwired: 1 in, 2 out]
                  }
                  frame #1 {
                    n1335 = for {
                      N: 40 -> [_]
                      tunnel: w1706 -> [w1713]
                      i -> [w1708]
                      n1336 = Compound Arithmetic op=ADD(0 ("值"), w1708) -> (w1710:i32)
                      n1337 = Bundle(w1710, 0) -> (w1712:cluster{i32, i32})  [unwired: 1 out]
                      n1338 = property class="Tbl (严格)"(reference=w1713, "Active Cell"=w1712, "Cell BG Color"=u32 16448250) -> ()  [unwired: 1 in, 2 out]
                    }
                  }
                  frame #2 {
                    n1339 = for {
                      N: 1 -> [_]
                      tunnel: w1715 -> [w1720]
                      i -> [w1716]
                      n1340 = Bundle(w1716, 0) -> (w1719:cluster{i32, i32})  [unwired: 1 out]
                      n1341 = property class="Tbl (严格)"(reference=w1720, "Active Cell"=w1719, "Cell BG Color"=u32 6618880) -> ()  [unwired: 1 in, 2 out]
                    }
                  }
                }
                n1342 = Select(t=0, s=w1689, f=1) -> (s? t:f=w1688:i32)
                n1343 = property on="项目信息 2" class="Tbl (严格)"("Disabled"=w1688) -> ()  [unwired: 2 in, 2 out]
                n1344 = property on="加热控制参数" class="Clust (严格)"("Disabled"=2) -> ()  [unwired: 2 in, 2 out]
                n1345 = global read "功能码全局.vi" "15"() -> (w1695:bool[])
                n1346 = Index Array(array=w1695, index #1=0 ("索引"), index #2=4 ("索引")) -> (element #1=w1693:bool, element #2=w1692:bool)
                n1347 = Not(x=w1686) -> (.not. x?=w1699:bool)
              }
              frame "通道电压节数" {
                w1721 = FALSE ("1 6")
                n1348 = property on="从板号" class="DigNum (严格)"("NumText.BGColor"=u32 16777215) -> ()  [unwired: 2 in, 2 out]
                n1349 = control-ref of="项目信息 2"() -> (w1732:refnum<vi>)
                n1350 = stacked-sequence {
                  tunnel: w1732 -> [w1739 w1741 w1750]
                  frame #0 {
                    n1351 = Bundle(22, 0) -> (w1738:cluster{i32, i32})  [unwired: 1 out]
                    n1352 = property class="Tbl (严格)"(reference=w1739, "Index Values"=w1738) -> ()  [unwired: 1 in, 2 out]
                  }
                  frame #1 {
                    n1353 = for {
                      N: 40 -> [_]
                      tunnel: w1741 -> [w1748]
                      i -> [w1743]
                      n1354 = Compound Arithmetic op=ADD(0 ("值"), w1743) -> (w1745:i32)
                      n1355 = Bundle(w1745, 0) -> (w1747:cluster{i32, i32})  [unwired: 1 out]
                      n1356 = property class="Tbl (严格)"(reference=w1748, "Active Cell"=w1747, "Cell BG Color"=u32 16448250) -> ()  [unwired: 1 in, 2 out]
                    }
                  }
                  frame #2 {
                    n1357 = for {
                      N: 5 -> [_]
                      tunnel: w1750 -> [w1757]
                      i -> [w1753]
                      n1358 = Add(x=22, y=w1753) -> (x+y=w1752:i32)
                      n1359 = Bundle(w1752, 0) -> (w1756:cluster{i32, i32})  [unwired: 1 out]
                      n1360 = property class="Tbl (严格)"(reference=w1757, "Active Cell"=w1756, "Cell BG Color"=u32 6618880) -> ()  [unwired: 1 in, 2 out]
                    }
                  }
                }
                n1361 = Select(t=0, s=w1724, f=1) -> (s? t:f=w1723:i32)
                n1362 = property on="项目信息 2" class="Tbl (严格)"("Disabled"=w1723) -> ()  [unwired: 2 in, 2 out]
                n1363 = property on="加热控制参数" class="Clust (严格)"("Disabled"=2) -> ()  [unwired: 2 in, 2 out]
                n1364 = global read "功能码全局.vi" "15"() -> (w1730:bool[])
                n1365 = Index Array(array=w1730, index #1=1 ("索引"), index #2=5 ("索引")) -> (element #1=w1728:bool, element #2=w1727:bool)
                n1366 = Not(x=w1721) -> (.not. x?=w1734:bool)
              }
              frame "保险位置" {
                w1758 = FALSE ("1 6")
                n1367 = control-ref of="项目信息 2"() -> (w1769:refnum<vi>)
                n1368 = stacked-sequence {
                  tunnel: w1769 -> [w1776 w1778 w1787]
                  frame #0 {
                    n1369 = Bundle(0, 0) -> (w1775:cluster{i32, i32})  [unwired: 1 out]
                    n1370 = property class="Tbl (严格)"(reference=w1776, "Index Values"=w1775) -> ()  [unwired: 1 in, 2 out]
                  }
                  frame #1 {
                    n1371 = for {
                      N: 40 -> [_]
                      tunnel: w1778 -> [w1785]
                      i -> [w1781]
                      n1372 = Add(x=2, y=w1781) -> (x+y=w1780:i32)
                      n1373 = Bundle(w1780, 0) -> (w1784:cluster{i32, i32})  [unwired: 1 out]
                      n1374 = property class="Tbl (严格)"(reference=w1785, "Active Cell"=w1784, "Cell BG Color"=u32 16448250) -> ()  [unwired: 1 in, 2 out]
                    }
                  }
                  frame #2 {
                    n1375 = for {
                      N: 20 -> [_]
                      tunnel: w1787 -> [w1794]
                      i -> [w1790]
                      n1376 = Add(x=2, y=w1790) -> (x+y=w1789:i32)
                      n1377 = Bundle(w1789, 0) -> (w1793:cluster{i32, i32})  [unwired: 1 out]
                      n1378 = property class="Tbl (严格)"(reference=w1794, "Active Cell"=w1793, "Cell BG Color"=u32 6618880) -> ()  [unwired: 1 in, 2 out]
                    }
                  }
                }
                n1379 = property on="从板号" class="DigNum (严格)"("NumText.BGColor"=u32 16777215) -> ()  [unwired: 2 in, 2 out]
                n1380 = Select(t=0, s=w1761, f=1) -> (s? t:f=w1760:i32)
                n1381 = property on="项目信息 2" class="Tbl (严格)"("Disabled"=w1760) -> ()  [unwired: 2 in, 2 out]
                n1382 = property on="加热控制参数" class="Clust (严格)"("Disabled"=2) -> ()  [unwired: 2 in, 2 out]
                n1383 = global read "功能码全局.vi" "15"() -> (w1767:bool[])
                n1384 = Index Array(array=w1767, index #1=2 ("索引"), index #2=6 ("索引")) -> (element #1=w1765:bool, element #2=w1764:bool)
                n1385 = Not(x=w1758) -> (.not. x?=w1771:bool)
              }
              frame "温度个数" {
                w1795 = FALSE ("1 6")
                n1386 = control-ref of="项目信息 2"() -> (w1806:refnum<vi>)
                n1387 = stacked-sequence {
                  tunnel: w1806 -> [w1813 w1814 w1824]
                  frame #0 {
                    n1388 = Bundle(0, 0) -> (w1812:cluster{i32, i32})  [unwired: 1 out]
                    n1389 = property class="Tbl (严格)"(reference=w1813, "Index Values"=w1812) -> ()  [unwired: 1 in, 2 out]
                  }
                  frame #1 {
                    n1390 = for {
                      N: 40 -> [_]
                      tunnel: w1814 -> [w1822]
                      i -> [w1817]
                      n1391 = Compound Arithmetic op=ADD(0 ("值"), w1817) -> (w1819:i32)
                      n1392 = Bundle(w1819, 0) -> (w1821:cluster{i32, i32})  [unwired: 1 out]
                      n1393 = property class="Tbl (严格)"(reference=w1822, "Active Cell"=w1821, "Cell BG Color"=u32 16448250) -> ()  [unwired: 1 in, 2 out]
                    }
                  }
                  frame #2 {
                    n1394 = for {
                      N: 1 -> [_]
                      tunnel: w1824 -> [w1831]
                      i -> [w1827]
                      n1395 = Add(x=1, y=w1827) -> (x+y=w1826:i32)
                      n1396 = Bundle(w1826, 0) -> (w1830:cluster{i32, i32})  [unwired: 1 out]
                      n1397 = property class="Tbl (严格)"(reference=w1831, "Active Cell"=w1830, "Cell BG Color"=u32 6618880) -> ()  [unwired: 1 in, 2 out]
                    }
                  }
                }
                n1398 = Select(t=0, s=w1798, f=1) -> (s? t:f=w1797:i32)
                n1399 = property on="项目信息 2" class="Tbl (严格)"("Disabled"=w1797) -> ()  [unwired: 2 in, 2 out]
                n1400 = property on="加热控制参数" class="Clust (严格)"("Disabled"=2) -> ()  [unwired: 2 in, 2 out]
                n1401 = property on="从板号" class="DigNum (严格)"("NumText.BGColor"=u32 16777215) -> ()  [unwired: 2 in, 2 out]
                n1402 = global read "功能码全局.vi" "15"() -> (w1804:bool[])
                n1403 = Index Array(array=w1804, index #1=3 ("索引"), index #2=7 ("索引")) -> (element #1=w1802:bool, element #2=w1801:bool)
                n1404 = Not(x=w1795) -> (.not. x?=w1808:bool)
              }
              frame "SOC过低", "电压不均衡", "电压过低", "电压过高", "温度不均衡", "温度过低", "温度过高", "一级故障阀值" {
                w1832 = FALSE ("1 6")
                n1405 = property on="从板号" class="DigNum (严格)"("NumText.BGColor"=u32 16777215) -> ()  [unwired: 2 in, 2 out]
                n1406 = Select(t=0, s=w1834, f=1) -> (s? t:f=w1835:i32)
                n1407 = property on="一级故障 6" class="Clust (严格)"("DisabledEnum"=w1835) -> ()  [unwired: 2 in, 2 out]
                n1408 = global read "功能码全局.vi" "18"() -> (w1841:bool[])
                n1409 = Index Array(array=w1841, index #1=2 ("索引"), index #2=5 ("索引")) -> (element #1=w1839:bool, element #2=w1838:bool)
                n1410 = Not(x=w1832) -> (.not. x?=w1843:bool)
              }
              frame "SOC过低(2)", "电压不均衡(2)", "电压过低(2)", "电压过高(2)", "二级故障阀值", "温度不均衡(2)", "温度过低(2)", "温度过高(2)" {
                w1845 = FALSE ("1 6")
                n1411 = property on="从板号" class="DigNum (严格)"("NumText.BGColor"=u32 16777215) -> ()  [unwired: 2 in, 2 out]
                n1412 = Select(t=0, s=w1848, f=1) -> (s? t:f=w1847:i32)
                n1413 = property on="一级故障 7" class="Clust (严格)"("DisabledEnum"=w1847) -> ()  [unwired: 2 in, 2 out]
                n1414 = global read "功能码全局.vi" "18"() -> (w1854:bool[])
                n1415 = Index Array(array=w1854, index #1=3 ("索引"), index #2=6 ("索引")) -> (element #1=w1852:bool, element #2=w1851:bool)
                n1416 = Not(x=w1845) -> (.not. x?=w1856:bool)
              }
              frame "SOC过低(3)", "电压不均衡(3)", "电压过低(3)", "电压过高(3)", "三级故障阀值", "温度不均衡(3)", "温度过低(3)", "温度过高(3)" {
                w1858 = FALSE ("1 6")
                n1417 = property on="从板号" class="DigNum (严格)"("NumText.BGColor"=u32 16777215) -> ()  [unwired: 2 in, 2 out]
                n1418 = Select(t=0, s=w1861, f=1) -> (s? t:f=w1860:i32)
                n1419 = property on="一级故障 8" class="Clust (严格)"("DisabledEnum"=w1860) -> ()  [unwired: 2 in, 2 out]
                n1420 = global read "功能码全局.vi" "18"() -> (w1867:bool[])
                n1421 = Index Array(array=w1867, index #1=4 ("索引"), index #2=7 ("索引")) -> (element #1=w1865:bool, element #2=w1864:bool)
                n1422 = Not(x=w1858) -> (.not. x?=w1869:bool)
              }
              frame "快换参数" {
                w1871 = FALSE ("1 6")
                n1423 = Select(t=0, s=w1892, f=1) -> (s? t:f=w1891:i32)
                n1424 = property on="电池组信息" class="Clust (严格)"("Disabled"=w1891) -> ()  [unwired: 2 in, 2 out]
                n1425 = property on="从板号" class="DigNum (严格)"("NumText.BGColor"=u32 16777215) -> ()  [unwired: 2 in, 2 out]
